vi "Identity Value.vi"(3 "Identity in":refnum<class "Identity.lvclass">) -> (1 "Value":string)   [LabVIEW 2020, in "Volatus.lvlib" / "Identity.lvclass"]
uses:
  Identity.lvclass
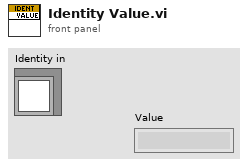
[diagram p1: front panel]
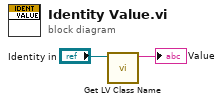
[diagram p0: block diagram]
diagram:
  n1 = call <vilib>:"Get LV Class Name.vi"("object"="Identity in") -> ("class name"=→"Value":string)  [unwired: 9 in, 1 out]
